vi "Input Validation.vi"(0 "Measurement Configuration":T1={"Quick Power Down"=FALSE, "Pin Name"=[], "Source Mode"=[], "Start Value"=[], "Target Value"=[], "Compliance Limit"=[], "Sense Mode"=[], "Default Ramp Rate"=[], "Ramp Rate"=[], "Start Delay"=[], "Relative To"=[], "Transient Response"=[], "Data Capture"=FALSE, "Power line frequency"=1} {"Power line frequency" items=["50 Hz", "60 Hz"]; "Start Value" format="%#_6p"; "Transient Response" items=["Slow", "Normal", "Fast"]; "Sense Mode" items=["Local Sense", "Remote Sense"]; "Relative To" items=["Power sequence start", "Previous source start", "Previous source end"]; "Target Value" format="%#_6p"; "Source Mode" items=["DC Voltage", "DC Current"]; "Start Delay" format="%#_6p"; "Compliance Limit" format="%#_6p"; "Ramp Rate" format="%#_6p"}, 5 "PowerUP?":bool, 11 "error in (no error)":errorcluster) -> (4 "Error":string[](array[string]), 15 "error out":errorcluster)   [LabVIEW 2024, in "devicePowerSequencerCoreLogic.lvlib"]
uses:
  devicePowerSequencerCoreLogic.lvlib
  Measurement Configuration.ctl
  controls/Source Mode.ctl
  controls/Sense Mode.ctl
  controls/Relative To.ctl
  controls/Transient Response.ctl
  controls/Power line frequency.ctl
  4ec2833f-6870-4676-a7e8-bb0dd69c3c6d.vi
  <vilib>/Utility/error.llb/Clear Errors.vi
  Form Error Message.vi/4da3fa3f-d6a2-4c6b-9c9c-fc44bca91f7b.vi
  <vilib>/Utility/error.llb/Error Cluster From Error Code.vi
  Device Power Sequencer.lvlib
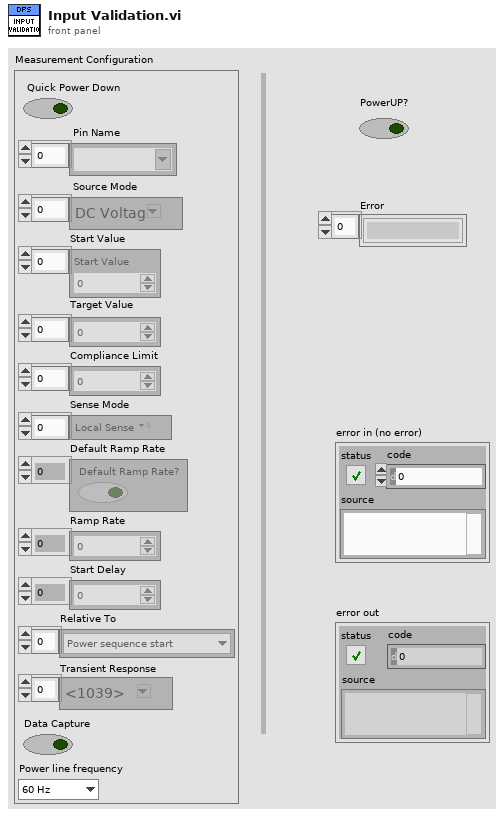
[diagram p1: front panel]
types:
  T1 = typedef "Device Power Sequencer.lvlib/Measurement Configuration.ctl" = cluster{"Quick Power Down":bool, "Pin Name":string[], "Source Mode":T2[], "Start Value":dbl[], "Target Value":dbl[], "Compliance Limit":dbl[], "Sense Mode":T3[], "Default Ramp Rate":bool[], "Ramp Rate":dbl[], "Start Delay":dbl[], "Relative To":T4[], "Transient Response":T5[], "Data Capture":bool, "Power line frequency":T6}
  T2 = typedef "Device Power Sequencer.lvlib/Source Mode.ctl" = i32
  T3 = typedef "Device Power Sequencer.lvlib/Sense Mode.ctl" = i32
  T4 = typedef "Device Power Sequencer.lvlib/Relative To.ctl" = u32
  T5 = typedef "Device Power Sequencer.lvlib/Transient Response.ctl" = i32
  T6 = typedef "Device Power Sequencer.lvlib/Power line frequency.ctl" = u32
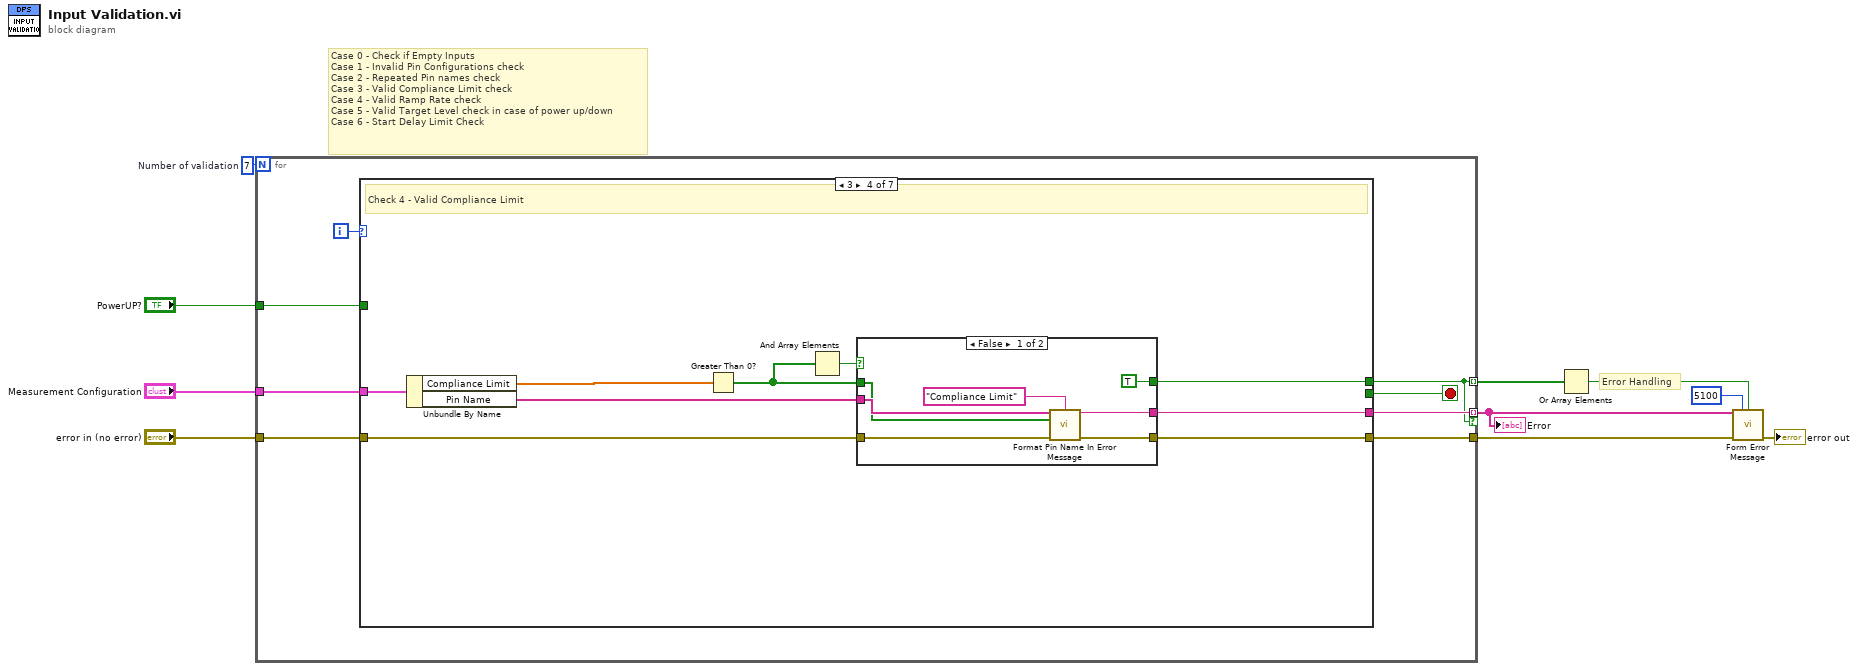
[diagram p0: block diagram]
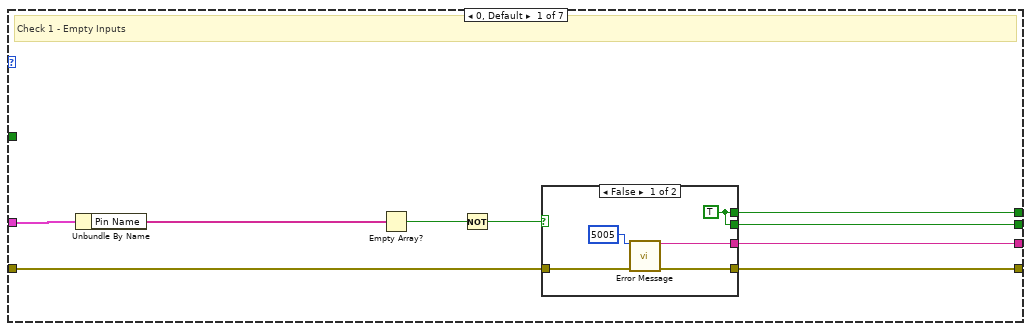
[diagram p2: hidden frame]
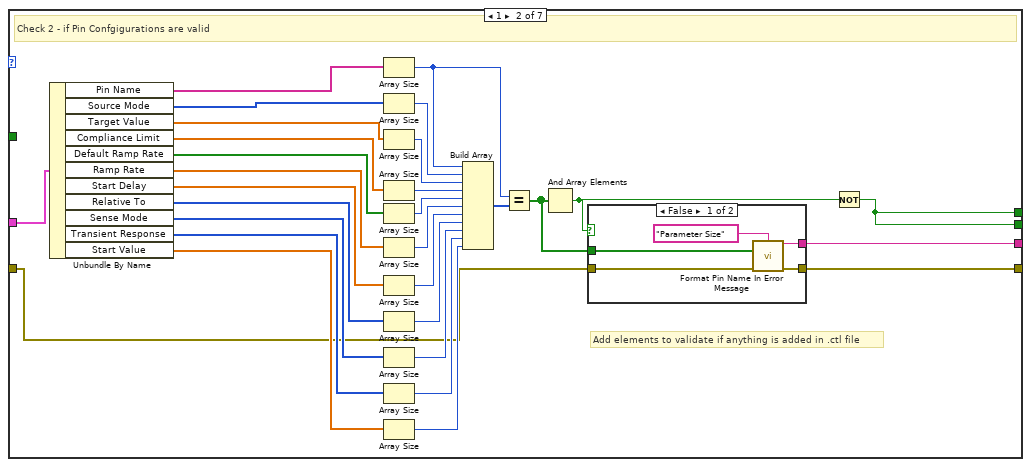
[diagram p4: hidden frame]
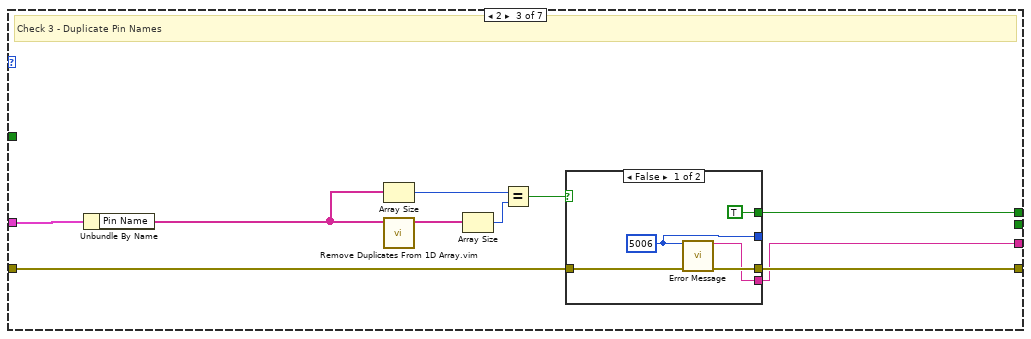
[diagram p6: hidden frame]
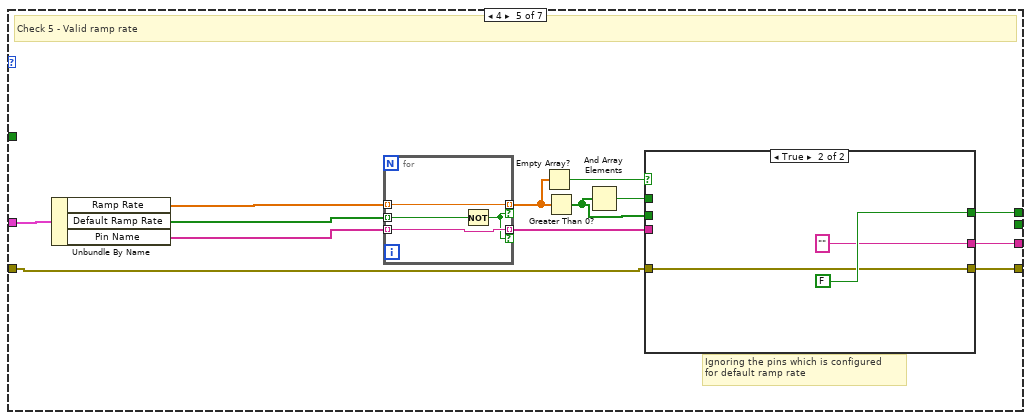
[diagram p9: hidden frame]
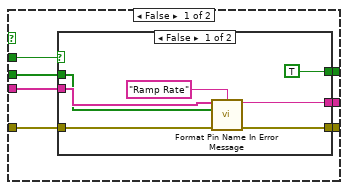
[diagram p10: hidden frame]
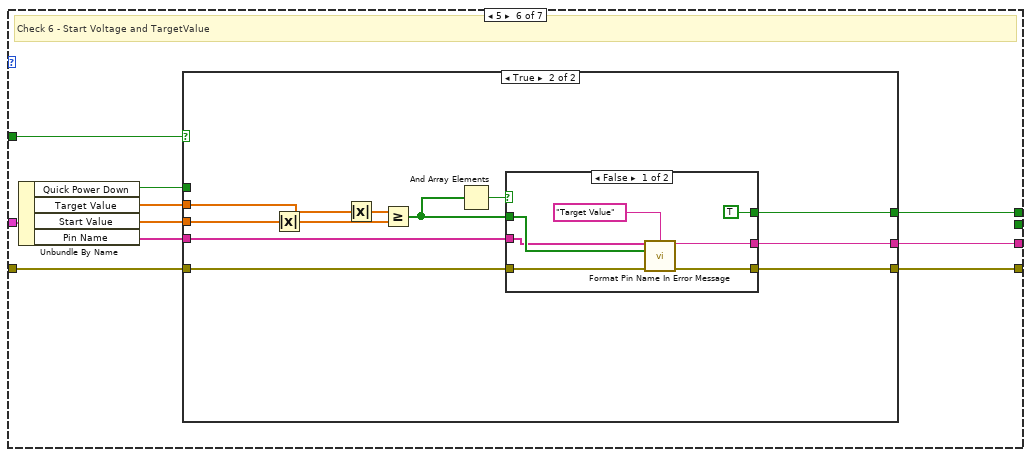
[diagram p12: hidden frame]
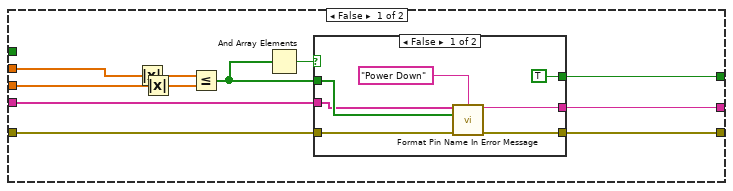
[diagram p13: hidden frame]
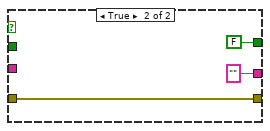
[diagram p14: hidden frame]
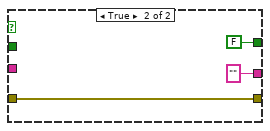
[diagram p15: hidden frame]
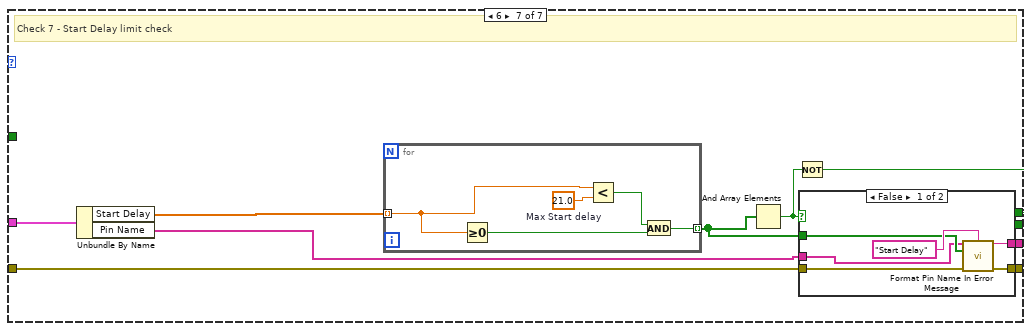
[diagram p16: hidden frame]
diagram:
  w10 = 7  # Number of validation
  # "Error Handling"
  # "Case 0 - Check if Empty Inputs\nCase 1 - Invalid Pin Configurations check\nCase 2 - Repeated Pin names check\nCase 3 - Valid Compliance Limit check\nCase 4 - Valid Ramp Rate check\nCase 5 - Valid Target Level check in case of power up/down \nCase 6 - Start Delay Limit Check"
  n1 = for {
    N: w10 -> [_]
    tunnel: "Measurement Configuration" -> [w18]
    tunnel: "error in (no error)" -> [w17]
    tunnel: [w15] -> w2 mode=indexing if=w13
    tunnel: [w16] -> w6
    tunnel: [w13] -> w7 mode=indexing
    tunnel: "PowerUP?" -> [w11]
    i -> [w12]
    stop <- w14 stop-if-true
    n2 = case shown="3" w12 {
      tunnel: w17 -> [w26 w35 w78 w94 w113 w145 w196]
      tunnel: [w25 w34 w77 w93 w112 w144 w194] -> w16
      tunnel: w18 -> [w27 w63 w79 w92 w115 w147 w198]
      tunnel: [w24 w37 w70 w91 w110 w143 w193] -> w15
      tunnel: [w23 w50 w71 w90 w111 w142 w192] -> w13
      tunnel: [w22 w50 _ _ _ _ _] -> w14
      tunnel: w11 -> [_ _ _ _ _ w138 _]
      frame 0, Default {
        # "Check 1 - Empty Inputs"
        n3 = Unbundle By Name(w27) -> ("Pin Name"=w21:string[])
        n4 = Empty Array?(array=w21) -> (empty?=w20:bool)
        n5 = Not(x=w20) -> (.not. x?=w19:bool)
        n6 = case shown="False" w19 {
          tunnel: w26 -> [w32 w33]
          tunnel: [w31 w33] -> w25
          tunnel: [w30 _] -> w24
          tunnel: [w29 _] -> w23
          tunnel: [w29 _] -> w22
          frame False {
            w29 = TRUE
            n7 = call "Error Message.vi"("Error Code"=5005, "error in (no error)"=w32) -> ("Error Message"=w30:string, "error out"=w31:errorcluster)  [unwired: 11 in, 1 out]
          }
          frame True {
            # "Check Passed"
          }
        }
      }
      frame 1 {
        # "Add elements to validate if anything is added in .ctl file"
        # "Check 2 - if Pin Confgigurations are valid"
        n8 = Unbundle By Name(w63) -> ("Pin Name"=w62:string[], "Source Mode"=w61:T2[], "Target Value"=w60:dbl[], "Compliance Limit"=w59:dbl[], "Default Ramp Rate"=w58:bool[], "Ramp Rate"=w57:dbl[], "Start Delay"=w56:dbl[], "Relative To"=w55:T4[], "Sense Mode"=w47:T3[], "Transient Response"=w43:T5[], "Start Value"=w42:dbl[])
        n9 = Array Size(array=w62) -> (size(s)=w39:i32)
        n10 = Array Size(array=w61) -> (size(s)=w54:i32)
        n11 = Array Size(array=w60) -> (size(s)=w53:i32)
        n12 = Array Size(array=w59) -> (size(s)=w52:i32)
        n13 = Array Size(array=w58) -> (size(s)=w48:i32)
        n14 = Array Size(array=w57) -> (size(s)=w49:i32)
        n15 = Array Size(array=w56) -> (size(s)=w51:i32)
        n16 = Array Size(array=w55) -> (size(s)=w45:i32)
        n17 = Array Size(array=w47) -> (size(s)=w44:i32)
        n18 = Array Size(array=w43) -> (size(s)=w41:i32)
        n19 = Array Size(array=w42) -> (size(s)=w40:i32)
        n20 = Build Array(w39, w54, w53, w52, w48, w49, w51, w45, w44, w41, w40) -> (w46:i32[])
        n21 = Equal?(x=w39, y=w46) -> (x = y?=w38:bool[])
        n22 = And Array Elements(Boolean array=w38) -> (logical AND=w36:bool)
        n23 = case shown="False" w36 {
          tunnel: w38 -> [w68 _]
          tunnel: [w67 _] -> w37
          tunnel: w35 -> [w65 w69]
          tunnel: [w64 w69] -> w34
          frame False {
            n24 = call "Format Pin Name In Error Message.vi"("Parameter Name"="Parameter Size", "Error[]"=w68, "error in"=w65) -> ("Error Message"=w67:string, "error out"=w64:errorcluster)  [unwired: 11 in]
          }
          frame True {
            # "Check Passed"
          }
        }
        n25 = Not(x=w36) -> (.not. x?=w50:bool)
      }
      frame 2 {
        # "Check 3 - Duplicate Pin Names"
        n26 = Unbundle By Name(w79) -> ("Pin Name"=w75:string[])
        n27 = Array Size(array=w75) -> (size(s)=w74:i32)
        n28 = call "Remove Duplicates From 1D Array.vim"("array"=w75) -> ("array with duplicates removed"=w76:string[])  [unwired: 10 in]
        n29 = Array Size(array=w76) -> (size(s)=w73:i32)
        n30 = Equal?(x=w74, y=w73) -> (x = y?=w72:bool)
        n31 = case shown="False" w72 {
          tunnel: w78 -> [w84 w85]
          tunnel: [w82 w85] -> w77
          tunnel: [TRUE _] -> w71
          tunnel: [w81 _] -> w70
          tunnel: [w80 _] -> _
          frame False {
            w80 = 5006 ("Error Code")
            n32 = call "Error Message.vi"("Error Code"=w80, "error in (no error)"=w84) -> ("Error Message"=w81:string, "error out"=w82:errorcluster)  [unwired: 11 in, 1 out]
          }
          frame True {
            # "Check Passed"
          }
        }
      }
      frame 3 {
        # "Check 4 - Valid Compliance Limit"
        n33 = Unbundle By Name(w92) -> ("Compliance Limit"=w87:dbl[], "Pin Name"=w88:string[])
        n34 = Greater Than 0?(x=w87) -> (x > 0?=w86:bool[])
        n35 = And Array Elements(Boolean array=w86) -> (logical AND=w89:bool)
        n36 = case shown="False" w89 {
          tunnel: w94 -> [w100 w102]
          tunnel: [w99 w102] -> w93
          tunnel: [w96 _] -> w91
          tunnel: [TRUE _] -> w90
          tunnel: w88 -> [w98 _]
          tunnel: w86 -> [w97 _]
          frame False {
            n37 = call "Format Pin Name In Error Message.vi"("Pin Name"=w98, "Parameter Name"="Compliance Limit", "Error[]"=w97, "error in"=w100) -> ("Error Message"=w96:string, "error out"=w99:errorcluster)  [unwired: 10 in]
          }
          frame True {
            # "Check Passed"
          }
        }
      }
      frame 4 {
        # "Ignoring the pins which is configured \nfor default ramp rate"
        # "Check 5 - Valid ramp rate"
        n38 = Unbundle By Name(w115) -> ("Ramp Rate"=w109:dbl[], "Default Ramp Rate"=w106:bool[], "Pin Name"=w105:string[])
        n39 = for {
          tunnel: w109 -> [w119] mode=indexing
          tunnel: [w119] -> w108 mode=indexing if=w116
          tunnel: w106 -> [w118] mode=indexing
          tunnel: w105 -> [w117] mode=indexing
          tunnel: [w117] -> w104 mode=indexing if=w116
          n40 = Not(x=w118) -> (.not. x?=w116:bool)
        }
        n41 = Empty Array?(array=w108) -> (empty?=w107:bool)
        n42 = Greater Than 0?(x=w108) -> (x > 0?=w103:bool[])
        n43 = And Array Elements(Boolean array=w103) -> (logical AND=w114:bool)
        n44 = case shown="True" w107 {
          tunnel: w114 -> [w126 _]
          tunnel: w113 -> [w125 w136]
          tunnel: [w124 w136] -> w112
          tunnel: [w123 FALSE] -> w111
          tunnel: [w122 "" ("Error Message")] -> w110
          tunnel: w104 -> [w121 _]
          tunnel: w103 -> [w120 _]
          frame False {
            n45 = case shown="False" w126 {
              tunnel: w125 -> [w129 w134]
              tunnel: [w128 w134] -> w124
              tunnel: [TRUE _] -> w123
              tunnel: [w127 _] -> w122
              tunnel: w121 -> [w131 _]
              tunnel: w120 -> [w130 _]
              frame False {
                n46 = call "Format Pin Name In Error Message.vi"("Pin Name"=w131, "Parameter Name"="Ramp Rate", "Error[]"=w130, "error in"=w129) -> ("Error Message"=w127:string, "error out"=w128:errorcluster)  [unwired: 10 in]
              }
              frame True {
                # "Check Passed"
              }
            }
          }
          frame True {
          }
        }
      }
      frame 5 {
        # "Check 6 - Start Voltage and TargetValue"
        n47 = Unbundle By Name(w147) -> ("Quick Power Down"=w139:bool, "Target Value"=w146:dbl[], "Start Value"=w141:dbl[], "Pin Name"=w140:string[])
        n48 = case shown="True" w138 {
          tunnel: w146 -> [w153 w179]
          tunnel: w145 -> [w155 w178]
          tunnel: [w157 w177] -> w144
          tunnel: [w158 w176] -> w143
          tunnel: [w156 w175] -> w142
          tunnel: w141 -> [w154 w174]
          tunnel: w140 -> [w152 w173]
          tunnel: w139 -> [_ _]
          frame False {
            n49 = Absolute Value(x=w153) -> (abs(x)=w148:dbl[])
            n50 = Absolute Value(x=w154) -> (abs(x)=w149:dbl[])
            n51 = Less Or Equal?(x=w148, y=w149) -> (x <= y?=w150:bool[])
            n52 = And Array Elements(Boolean array=w150) -> (logical AND=w151:bool)
            n53 = case shown="False" w151 {
              tunnel: w155 -> [w165 w168]
              tunnel: [w164 w168] -> w157
              tunnel: [w163 "" ("Error Message")] -> w158
              tunnel: [TRUE FALSE] -> w156
              tunnel: w150 -> [w161 _]
              tunnel: w152 -> [w160 _]
              frame False {
                n54 = call "Format Pin Name In Error Message.vi"("Pin Name"=w160, "Parameter Name"="Power Down", "Error[]"=w161, "error in"=w165) -> ("Error Message"=w163:string, "error out"=w164:errorcluster)  [unwired: 10 in]
              }
              frame True {
              }
            }
          }
          frame True {
            n55 = Absolute Value(x=w174) -> (abs(x)=w169:dbl[])
            n56 = Absolute Value(x=w179) -> (abs(x)=w170:dbl[])
            n57 = Greater Or Equal?(x=w170, y=w169) -> (x >= y?=w171:bool[])
            n58 = And Array Elements(Boolean array=w171) -> (logical AND=w172:bool)
            n59 = case shown="False" w172 {
              tunnel: w178 -> [w186 w189]
              tunnel: [w185 w189] -> w177
              tunnel: [w184 "" ("Error Message")] -> w176
              tunnel: [TRUE FALSE] -> w175
              tunnel: w171 -> [w182 _]
              tunnel: w173 -> [w181 _]
              frame False {
                n60 = call "Format Pin Name In Error Message.vi"("Pin Name"=w181, "Parameter Name"="Target Value", "Error[]"=w182, "error in"=w186) -> ("Error Message"=w184:string, "error out"=w185:errorcluster)  [unwired: 10 in]
              }
              frame True {
              }
            }
          }
        }
      }
      frame 6 {
        # "Check 7 - Start Delay limit check"
        n61 = Unbundle By Name(w198) -> ("Start Delay"=w197:dbl[], "Pin Name"=w190:string[])
        n62 = for {
          tunnel: w197 -> [w202] mode=indexing
          tunnel: [w199] -> w191 mode=indexing
          w203 = 21.0  # Max Start delay
          n63 = Greater Or Equal To 0?(x=w202) -> (x >= 0?=w201:bool)
          n64 = Less?(x=w202, y=w203) -> (x < y?=w200:bool)
          n65 = And(x=w200, y=w201) -> (x .and. y?=w199:bool)
        }
        n66 = And Array Elements(Boolean array=w191) -> (logical AND=w195:bool)
        n67 = Not(x=w195) -> (.not. x?=w192:bool)
        n68 = case shown="False" w195 {
          tunnel: w196 -> [w208 w210]
          tunnel: [w207 w210] -> w194
          tunnel: [w206 _] -> w193
          tunnel: w191 -> [w205 _]
          tunnel: w190 -> [w204 _]
          frame False {
            n69 = call "Format Pin Name In Error Message.vi"("Pin Name"=w204, "Parameter Name"="Start Delay", "Error[]"=w205, "error in"=w208) -> ("Error Message"=w206:string, "error out"=w207:errorcluster)  [unwired: 10 in]
          }
          frame True {
            # "Check Passed"
          }
        }
      }
    }
  }
  "Error" <- w2
  n70 = Or Array Elements(Boolean array=w7) -> (logical OR=w4:bool)
  n71 = call "Form Error Message.vi"("Error Message"=w2, "error code (0)"=5100, "Error?"=w4, "error in (no error)"=w6) -> ("error out"=→"error out":errorcluster)  [unwired: 11 in]
